vi "SetTrig.vi"(8 "error in (no error)":errorcluster, 9 "TX trigger options":T1, 10 "Port":string(combo), 11 "reference in":refnum<class "niMmWave_Transceiver.lvclass">) -> (0 "error out":errorcluster, 3 "reference out":refnum<class "niMmWave_Transceiver.lvclass">)   [LabVIEW 2019, in "niMmWave_Transceiver.lvclass"]
uses:
  niMmWave_Transceiver.lvclass
  Low-level/TypeDefs/TX trigger config.ctl
  FPGA/SubVIs/Utility/FPGA driver trigger source.ctl
  FPGA/SubVIs/Utility/FPGA driver trigger destination.ctl
  FPGA/SubVIs/Utility/FPGA Utility.lvlib
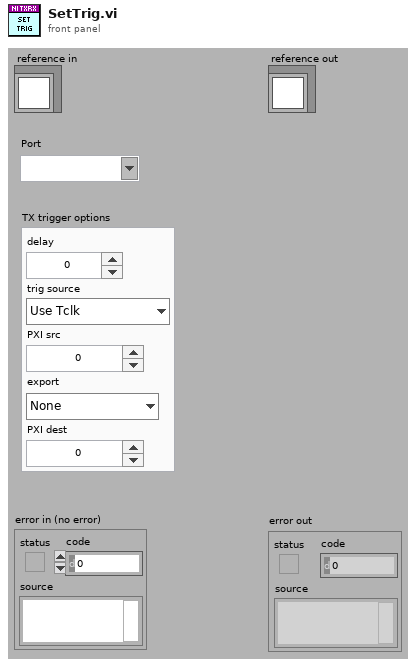
[diagram p1: front panel]
types:
  T1 = typedef "TX trigger config.ctl" = cluster{"delay":dbl, "trig source":T2, "PXI src":i32, "export":T3, "PXI dest":i32}
  T2 = typedef "FPGA Utility.lvlib/FPGA driver trigger source.ctl" = enum16{"Use Tclk", "PXI_Trig", "Aurora RX trig"}
  T3 = typedef "FPGA Utility.lvlib/FPGA driver trigger destination.ctl" = enum16{"None", "Source trig", "Synced trig", "Delayed sync"}
  T4 = typedef "niMmWave_Transceiver.lvclass/ObjectAttributesRef.ctl" = refnum<data-value>
  T5 = typedef "niMmWave_Transceiver.lvclass/ObjectAttributes.ctl" = cluster{"session":T6[], "HW.RX resources":T20, "RF config":T21, "RX trigger options":T1, "TX trigger options":T1, "RX samples":i32, "Downloaded Bursts":map{string, T22}, "TX Fs":dbl, "RX Fs":dbl, "burst sequence":string[]}
  T6 = typedef "Session.ctl" = cluster{"3620 session":refnum<queue>, "tx baseband session":T7, "rx baseband session":T15, "tx gain (dB)":dbl, "rx gain (dB)":dbl, "hardware configuration":T16, "gain ranging":T18[], "pxi trigger bus information":T19}
  T7 = typedef "Tx Baseband Session.ctl" = cluster{"3610 session":T8, "7902 reference":T14}
  T8 = typedef "ni3610_and_ni3630_Driver_Lib.lvlib/Main Settings.ctl" = cluster{"VISA resource name":refnum<visa-resource-name>, "Address Space":T9, "window_offset":u32, "register_addresses":T10, "required_MM_fpga_version":cluster{"signature":u32, "hardware":u32, "current revision":u32, "oldest revision":u32}, "CPLD Oldest Compat Version ":cluster{"hardware":u32, "CPLD firmware":u32}, "MM_FPGA_image_location":string, "is_init":bool, "card_type":T11, "DacLmkConfigFileName":string, "AdcLmkConfigFileName":string, "AdcConfigFileName":string, "DacConfigFileName_RevA":string, "DacConfigFileName_RevB":string, "Mulde hardware revision":u8, "bypass DAC PLL\n":bool, "IQ Card Revision":T12, "board capability":T13}
  T9 = typedef "VISA Register Access Address Space.ctl" = u16
  T10 = typedef "ni3610_and_ni3630_Driver_Lib.lvlib/Register Adresses.ctl" = cluster{"MM based Registers":cluster{"Revision":u32, "OldestCompatRev":u32, "signature":u32, "scratch":u32, "LedControl":u32, "BoardHwRev":u32, "BoardControl":u32, "ThermalStatus":u32, "BasebandStatus":u32, "BasebandControl":u32, "BasebandAuxSetup":u32, "BasebandAuxStatus":u32, "LmkSyncOutSetup":u32, " AdcSyncOutSetup":u32, " InjSyncOutSetup":u32, " PxiTrig0OutSetup":u32, " PxiTrig1OutSetup":u32, " PxiTrig2OutSetup":u32, " PxiTrig3OutSetup":u32, " PxiTrig4OutSetup":u32, " PxiTrig5OutSetup":u32, " PxiTrig6OutSetup":u32, " PxiTrig7OutSetup":u32}, "CPLD based Registers":cluster{"SlaveSignature":u32, "SlaveRevision":u32, "SlaveOldestCompatRev":u32, "SlaveScratch":u32, "SlaveSetup":u32, "SlaveStatus":u32, "IDacReg_offset":u32, "LMKRegGrp0_offset":u32, "QDacReg_offset":u32, "BrdTempSensorVal":u32, "TempSensorPowerDown":u32, "GPIOReg_offset":u32, "IAdcReg_offset":u32, "QAdcReg_offset":u32, "LMKRegGrp1_offset":u32, "QadcTempSensorVal":u32, "IadcTempSensorVal":u32, "RevisionReg":u32, "VcxoReg":u32, "CpldStatusReg":u32, "PowerReg":u32, "VBiasEnReg":u32, "ExtRefOeReg":u32, "QdacCtrlReg":u32, "QdacStatusReg":u32, "IdacCtrlReg":u32, "IdacStatusReg":u32, "QdacJtagIn":u32, "QdacJtagOut":u32, "IdacJtagIn":u32, "IdacJtagOut":u32, "IqDcSetupReg":u32, "QadcStatusReg":u32, "IadcStatusReg":u32, "BrdSetupReg":u32, "IqDcRevisionReg":u32, "PllStatusReg":u32, "EndpointScratchReg":u32, "AdcSyncCfgReg":u32, "IqCardOpampReg":u32}, "CPLD Register Offset":u32, "MM  Register Offset":u32, " PxiTrig0OutSetup":u32}
  T11 = typedef "ni3610_and_ni3630_Driver_Lib.lvlib/Base Card Type.ctl" = enum16{"unspecified", "ADC", "DAC"}
  T12 = typedef "ni3610_and_ni3630_Driver_Lib.lvlib/IQ Card Revision.ctl" = enum16{"RevA", "RevB", "RevC", "RevD"}
  T13 = typedef "ni3610_and_ni3630_Driver_Lib.lvlib/Board Capability.ctl" = cluster{"baseband sync":enum16{"no baseband sync", "baseband sync"}}
  T14 = typedef "Blank FPGA Reference.ctl" = refnum<k20>
  T15 = typedef "Rx Baseband Session.ctl" = cluster{"3630 session":T8, "7902 reference":T14}
  T16 = typedef "Hardware Configuration.ctl" = cluster{"direction":T17, "baseband only":bool}
  T17 = typedef "Direction.ctl" = enum16{"Transceiver", "Receiver", "Transmitter"}
  T18 = typedef "Gain Ranging.ctl" = cluster{"gain ranging active scope":string, "gain ranging stream session":refnum<k20>}
  T19 = typedef "PXI Trigger Bus Info.ctl" = cluster{"chassis resource name":refnum<visa-resource-name>, "7902R (TX)":i16, "3610 (TX)":i16, "3620 (IF)":i16, "3630 (RX)":i16, "7902R (RX)":i16}
  T20 = typedef "mmWave HW Control.lvlib/HW TXRX resources cluster.ctl" = cluster{"TX_DAC":refnum<visa-resource-name>, "TX_FPGA":tag, "IF":tag, "RX_ADC":refnum<visa-resource-name>, "RX_FPGA":tag}
  T21 = typedef "mmWave HW Control.lvlib/HW TXRX RF config cluster.ctl" = cluster{"TX.Frequency":dbl, "TX.Gain":dbl, "TX.mmWave adapter":string, "RX.Frequency":dbl, "RX.Gain":dbl, "RX.mmWave adapter":string}
  T22 = typedef "niMmWave_Transceiver.lvclass/BurstInfo.ctl" = cluster{"starting addr":u32, "end addr":u32}
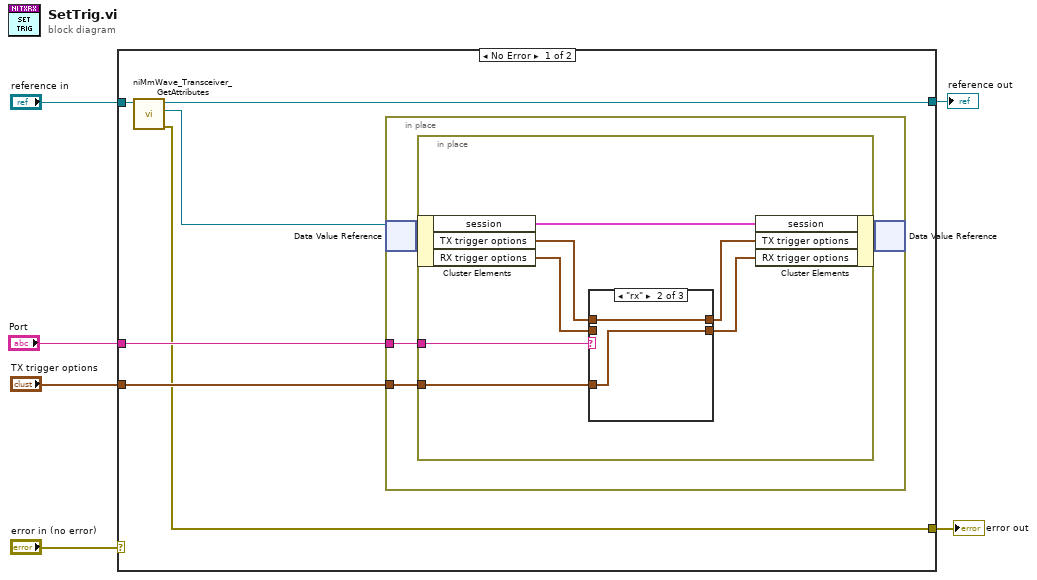
[diagram p0: block diagram]
diagram:
  n1 = case shown="No Error" "error in (no error)" {
    selector: "error in (no error)" -> [_ w31]
    tunnel: [w7 w31] -> w5
    tunnel: [w12 w30] -> w3
    tunnel: "reference in" -> [w11 w30]
    tunnel: "Port" -> [w9 _]
    tunnel: "TX trigger options" -> [w8 _]
    frame No Error {
      n2 = call "niMmWave_Transceiver_GetAttributes.vi"("reference in"=w11) -> ("error out"=w7:errorcluster, "attributes ref"=w10:T4, "reference out"=w12:refnum<class "niMmWave_Transceiver.lvclass">)  [unwired: 7 in, 1 out]
      n3 = in-place {
        in-place-border: w9 -> [w14]
        in-place-border: w8 -> [w13]
        n4 = in-place-dvr #1(w10) -> (w16:T5)  [unwired: 1 out]
        n5 = in-place {
          in-place-border: w14 -> [w22]
          in-place-border: w13 -> [w21]
          n6 = in-place-cluster #2(w16) -> ("session"=w23:T6[], "TX trigger options"=w20:T1, "RX trigger options"=w19:T1)
          n7 = case shown="\"rx\"" w22 {
            tunnel: w20 -> [_ w27 w29]
            tunnel: w21 -> [w24 w26 _]
            tunnel: w19 -> [w25 _ w28]
            tunnel: [w24 w27 w29] -> w18
            tunnel: [w25 w26 w28] -> w17
            frame "tx" {
            }
            frame "rx" {
            }
            frame Default {
            }
          }
          n8 = in-place-cluster #2("session"=w23, "TX trigger options"=w18, "RX trigger options"=w17) -> (w15:T5)
        }
        n9 = in-place-dvr #1(w15) -> ()  [unwired: 2 out]
      }
    }
    frame Error {
    }
  }
  "error out" <- w5
  "reference out" <- w3
